vi "Write My Data to HDF5.vi"(4 "Data":T1(array[cluster]), 5 "Comment":string, 7 "Time Stamp":timestamp, 8 "error in":errorcluster, 10 "Dataset Path":string, 11 "file path":path) -> (0 "error out":errorcluster)   [LabVIEW 2011]
uses:
  Users/Jason/Documents/lvhdf5/trunk/vi.lib/UPVI/lvhdf5/attribute.llb/LVH5A Operation.ctl
  <vilib>/Utility/miscctls.llb/LVRectTypeDef.ctl
  Users/Jason/Documents/lvhdf5/trunk/vi.lib/UPVI/lvhdf5/file.llb/LVH5F Operation.ctl
  Users/Jason/Documents/lvhdf5/trunk/vi.lib/UPVI/lvhdf5/dataset.llb/LVH5D Operation.ctl
  Users/Jason/Documents/lvhdf5/trunk/vi.lib/UPVI/lvhdf5/group.llb/H5G_obj_t.ctl
  Users/Jason/Documents/lvhdf5/trunk/vi.lib/UPVI/lvhdf5/identifier.llb/Not an HDF5 Refnum Constant.vi
  Users/Jason/Documents/lvhdf5/trunk/vi.lib/UPVI/lvhdf5/common.llb/To HDF5 Ref.vi
  Users/Jason/Documents/lvhdf5/trunk/vi.lib/UPVI/lvhdf5/attribute.llb/Write Multiple Attributes.vi
  Users/Jason/Documents/lvhdf5/trunk/vi.lib/UPVI/lvhdf5/file.llb/OpenCreateReplace HDF5 File.vi
  Users/Jason/Documents/lvhdf5/trunk/vi.lib/UPVI/lvhdf5/utility.llb/Select HDF5 Dialog.vi
  Users/Jason/Documents/lvhdf5/trunk/vi.lib/UPVI/lvhdf5/utility.llb/Select HDF5 Dialog (File and Object).vi
  Users/Jason/Documents/lvhdf5/trunk/vi.lib/UPVI/lvhdf5/dataset.llb/Simple H5Dwrite (Variant).vi
  Users/Jason/Documents/lvhdf5/trunk/vi.lib/UPVI/lvhdf5/dataset.llb/H5Dclose.vi
  Users/Jason/Documents/lvhdf5/trunk/vi.lib/UPVI/lvhdf5/file.llb/H5Fclose.vi
  Users/Jason/Documents/lvhdf5/trunk/vi.lib/UPVI/lvhdf5/dataset.llb/Write Dataset with Attributes.xnode
  Users/Jason/Documents/lvhdf5/trunk/vi.lib/UPVI/lvhdf5/library.llb/HDF5 Ref.ctl
  <vilib>/Utility/error.llb/Error Cluster From Error Code.vi
  Users/Jason/Documents/lvhdf5/trunk/vi.lib/UPVI/lvhdf5/dataset.llb/OpenCreateReplace Dataset by Element Type.vi
  Users/Jason/Documents/lvhdf5/trunk/vi.lib/UPVI/lvhdf5/dataspace.llb/H5Sselect_hyperslab.vi
  Users/Jason/Documents/lvhdf5/trunk/vi.lib/UPVI/lvhdf5/dataset.llb/H5Dwrite (Variant).vi
  Users/Jason/Documents/lvhdf5/trunk/vi.lib/UPVI/lvhdf5/dataset.llb/H5Dget_space.vi
  Users/Jason/Documents/lvhdf5/trunk/vi.lib/UPVI/lvhdf5/attribute.llb/private/LVH5AwriteWDTAttrs.vi
  Users/Jason/Documents/lvhdf5/trunk/vi.lib/UPVI/lvhdf5/dataspace.llb/H5Sclose.vi
  Users/Jason/Documents/lvhdf5/trunk/vi.lib/UPVI/lvhdf5/utility.llb/Select HDF5 Dialog (Object Only).vi
  <vilib>/Utility/VariantDataType/GetClusterInfo.vi
  <vilib>/Utility/VariantDataType/VariantType.lvlib
  <vilib>/Utility/VariantDataType/GetTypeInfo.vi
  Users/Jason/Documents/lvhdf5/trunk/vi.lib/UPVI/lvhdf5/attribute.llb/Cluster to Attribute Array.xnode
panel:
  in  "Good":bool
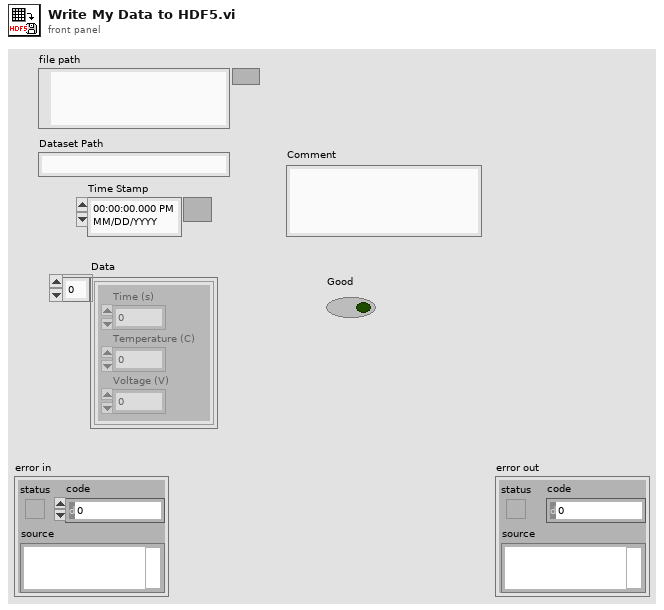
[diagram p1: front panel]
types:
  T1 = cluster{"Time (s)":dbl, "Temperature (C)":dbl, "Voltage (V)":dbl}[]
  T2 = typedef "LVH5A Operation.ctl" = enum16{"open", "replace", "create", "open or create", "create or replace", "create or replace with confirmation"}
  T3 = typedef "LVRectTypeDef.ctl" = cluster{"Left":i16, "Top":i16, "Right":i16, "Bottom":i16}
  T4 = cluster{"Behavior":enum32{"Invalid", "Default", "Floating", "Floating/Auto-Hide", "Modal"}, "Position":T3, "Center":bool, "Title":string}
  T5 = typedef "LVH5F Operation.ctl" = enum16{"open", "open or create", "create or replace", "create or replace (with confirmation)", "create", "open (read only)"}
  T6 = typedef "LVH5D Operation.ctl" = enum16{"open", "replace", "create", "open or create", "create or replace", "create or replace with confirmation"}
  T7 = typedef "H5G_obj_t.ctl" = i32
  T8 = cluster{"Object Types (any)":T7[], "Object Pattern":string}
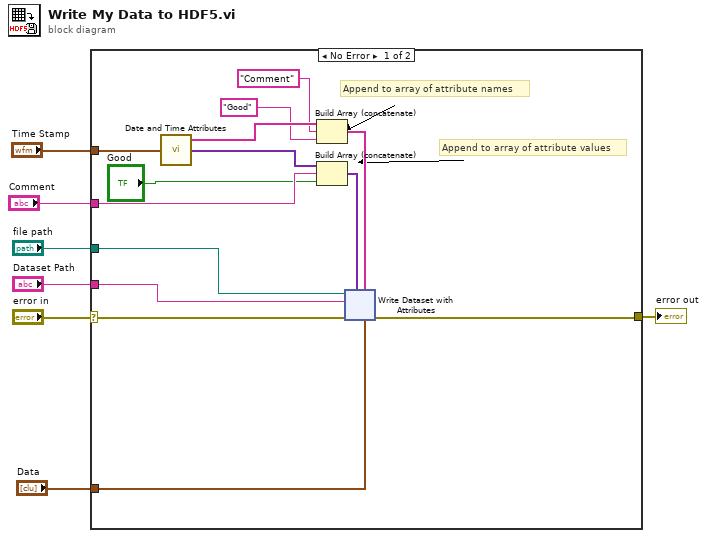
[diagram p0: block diagram]
diagram:
  n1 = case shown="No Error" "error in" {
    selector: "error in" -> [w12 w316]
    tunnel: "Data" -> [w21 _]
    tunnel: [w13 w316] -> w7
    tunnel: "file path" -> [w11 _]
    tunnel: "Time Stamp" -> [w20 _]
    tunnel: "Comment" -> [w16 _]
    tunnel: "Dataset Path" -> [w10 _]
    frame No Error {
      # "Append to array of attribute values"
      # "Append to array of attribute names"
      n2 = call "Date and Time Attributes.vi"("Timestamp (current)"=w20) -> ("Attribute Names"=w19:string[], "Attribute Values"=w17:variant[])  [unwired: 1 out]
      n3 = Build Array (concatenate)(w19, "Comment", "Good" ("element")) -> (w14:string[])
      n4 = Build Array (concatenate)(w17, w16, "Good") -> (w15:variant[])
      n5 = xnode "Write Dataset with Attributes"("Dataset Path"=w10, "error in (no error)"=w12, "HDF5 Path or Ref"=w11, "Attribute Name(s)"=w14, "Attribute Value(s)"=w15, "Data"=w21) -> ("error out"=w13:errorcluster)  [unwired: 2 in, 2 out]
    }
    frame Error {
      # "Wire previous error through"
    }
  }
  "error out" <- w7
